vi "ColorscaleIgor.vi"() -> ()   [LabVIEW 2020]
uses:
  <userlib>/LevyLab/Graph Utilities/graph_utilities.lvclass
  <userlib>/LevyLab/LV-Data/LV-Data.ITX/LV-Data.ITX.lvclass
panel:
  in  "path":path
  in  "Color Map":T1(ring)=enum."Viridis"
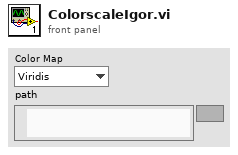
[diagram p1: front panel]
types:
  T1 = enum16{"Inferno", "Kindlmann", "Plasma", "Viridis", "LevyLab2010", "ColorCET...", "Custom..."}
  T2 = cluster{"2D Array":dbl[][], "X 1D Array":dbl[], "Y 1D Array":dbl[]}
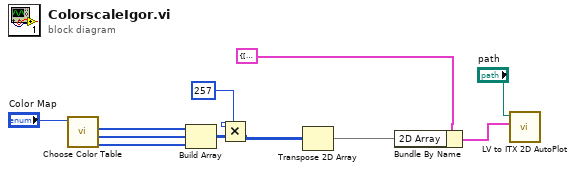
[diagram p0: block diagram]
diagram:
  n1 = call <userlib>:"Choose Color Table.vi"("Color Map"="Color Map") -> ("B []"=w9:u8[], "G []"=w10:u8[], "R []"=w11:u8[])  [unwired: 7 in, 1 out]
  n2 = Build Array(w11, w10, w9) -> (w7:u8[][])
  n3 = Multiply(x=257, y=w7) -> (x*y=w3:i32[][])
  n4 = Transpose 2D Array(2D array=w3) -> (transposed array=w1:i32[][])
  n5 = Bundle By Name(cluster=T2 {"2D Array"=[], "X 1D Array"=[], "Y 1D Array"=[]} ("2D, X, Y (Cluster)"), "2D Array"=w1) -> (w5:T2)
  n6 = call <userlib>:"LV to ITX 2D AutoPlot.vi"("2D, X, Y (Cluster)"=w5, "path"="path") -> ()  [unwired: 8 in, 2 out]
